vi "Init_Test.vi"(8 "error in (no error)":errorcluster caption="entrée d'erreur (pas d'erreur)", 11 "Print_Label en entrée":refnum<class "Get_SN_DB_AIS.lvclass">) -> (0 "error out":errorcluster caption="sortie d'erreur", 3 "Print_Label en sortie":refnum<class "Get_SN_DB_AIS.lvclass">)   [LabVIEW 2020, in "Library Test.lvlib" / "Get_SN_DB_AIS.lvclass"]
uses:
  Get_SN_DB_AIS.lvclass
  C:/Users/ngarcin/OneDrive - Altyor/Standard TB/Class/Test/Test (Default)/Test (Default).lvclass
  Commun VI/TypeDef/Commande Test/Commande Value Type.ctl
  Commun VI/TypeDef/Commande Test/Commande Type Test.ctl
  Test_Wtih_Instr/Test_With_Inst.lvclass
  Instrument/Instrument (Default)/Class Instrument (Default).lvclass
  Get_SN_DB_AIS.lvclass/Get_SN_DB_AIS.ctl
  Commun VI/Library Commun.lvlib
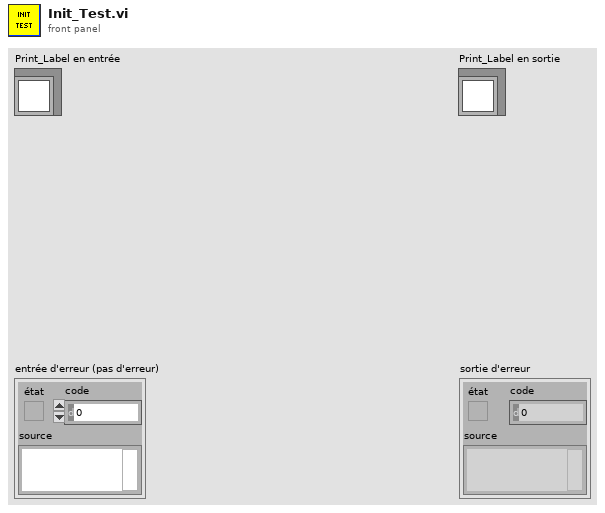
[diagram p1: front panel]
types:
  T1 = typedef "Library Commun.lvlib/Commande Type Test.ctl" = enum16{"Function", "Test", "Calculation"}
  T2 = typedef "Library Commun.lvlib/Commande Value Type.ctl" = enum16{"None", "String", "Number", "Timestamp", "Boolean", "Array"}
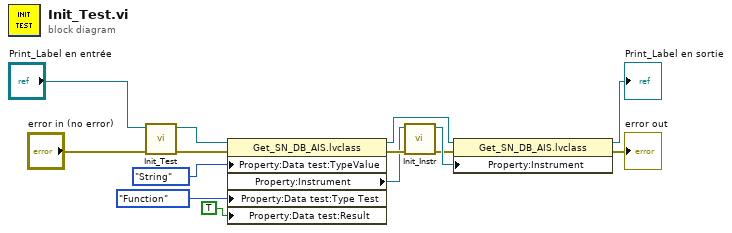
[diagram p0: block diagram]
diagram:
  n1 = call-parent "Init_Test.vi"("error in (no error)"="error in (no error)", "Test_With_Inst en entrée"="Print_Label en entrée") -> ("error out"=w11:errorcluster, "Test_With_Inst en sortie"=w12:refnum<class "Get_SN_DB_AIS.lvclass">)  [unwired: 8 in]
  n2 = property class="Get_SN_DB_AIS.lvclass"(reference=w12, error in=w11, "Property:Data test:TypeValue"=Commande_Value_Type."String" ("TypeValue"), "Property:Data test:Type Test"=Commande_Type_Test."Function" ("Type Test"), "Property:Data test:Result"=TRUE ("Result")) -> (reference out=w10:refnum<class "Get_SN_DB_AIS.lvclass">, error out=w5:errorcluster, "Property:Instrument"=w4:refnum<class "Class Instrument (Default).lvclass">)
  n3 = call-dynamic "Init_Instr.vi"("error in (no error)"=w5, "Class Instrument (Default) en entrée"=w4) -> ("error out"=w2:errorcluster, "Class Instrument (Default) en sortie"=w3:refnum<class "Class Instrument (Default).lvclass">)  [unwired: 8 in]
  n4 = property class="Get_SN_DB_AIS.lvclass"(reference=w10, error in=w2, "Property:Instrument"=w3) -> (reference out=→"Print_Label en sortie":refnum<class "Get_SN_DB_AIS.lvclass">, error out=→"error out":errorcluster)
